vi "PID Output_Buffer_Dbl_VIG.vi"(6 "Automatic":bool=TRUE, 7 "Operation":T1(ring)=enum."set manual data", 8 "error in":errorcluster, 11 "Numeric":dbl) -> (0 "error out":errorcluster, 3 "Numeric":dbl)   [LabVIEW 2018]
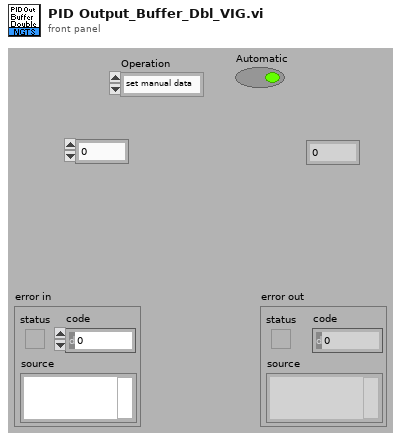
[diagram p1: front panel]
types:
  T1 = enum16{"get data", "set manual data", "set automatic data", "Set Mode", "initialize"}
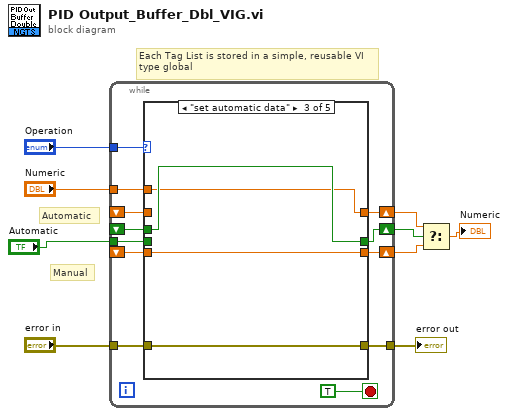
[diagram p0: block diagram]
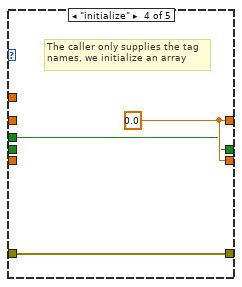
[diagram p4: hidden frame]
diagram:
  # "Automatic"
  # "Manual"
  # "Each Tag List is stored in a simple, reusable VI\ntype global"
  n1 = while {
    tunnel: "Operation" -> [w21]
    shift-right: [w19] -> w4
    shift-left: _ -> [w17]
    tunnel: "Numeric" -> [w18]
    tunnel: "error in" -> [w16]
    tunnel: [w15] -> w6
    shift-right: [w14] -> w3
    shift-left: _ -> [w13]
    shift-right: [w11] -> w1
    shift-left: _ -> [w12]
    tunnel: "Automatic" -> [w10]
    stop <- TRUE stop-if-true
    n2 = case shown="\"set automatic data\"" w21 {
      tunnel: [w25 w27 w31 w35 w40] -> w19
      tunnel: w18 -> [_ w28 w31 _ _]
      tunnel: w17 -> [w25 w27 _ _ w40]
      tunnel: w16 -> [w24 w29 w33 w36 w37]
      tunnel: [w24 w29 w33 w36 w37] -> w15
      tunnel: [w23 w28 w30 w35 w39] -> w14
      tunnel: w13 -> [w23 _ w30 _ w39]
      tunnel: w12 -> [w22 w26 w32 w34 _]
      tunnel: [w22 w26 w32 w34 w38] -> w11
      tunnel: w10 -> [_ _ _ _ w38]
      frame "get data", Default {
      }
      frame "set manual data" {
      }
      frame "set automatic data" {
      }
      frame "initialize" {
        w35 = 0.0 ("element")
        # "The caller only supplies the tag\nnames, we initialize an array"
      }
      frame "Set Mode" {
      }
    }
  }
  "error out" <- w6
  n3 = Select(t=w4, s=w1, f=w3) -> (s? t:f=→"Numeric":dbl)
